vi "Create Task Taking XML.vi"(8 "error in (no error)":errorcluster) -> (0 "error out":errorcluster, 3 "Take Task XML":string)   [LabVIEW 2012]
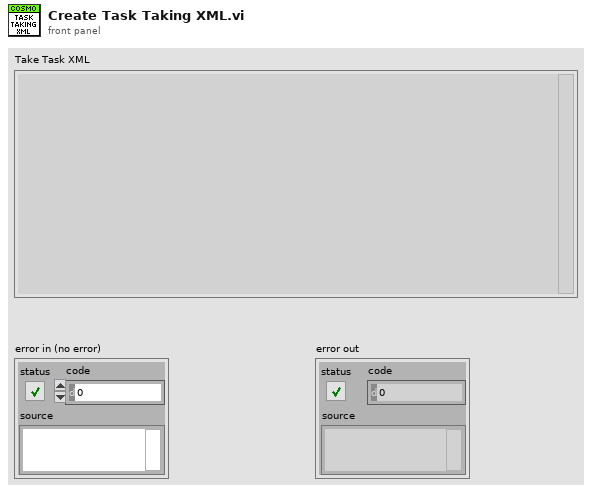
[diagram p1: front panel]
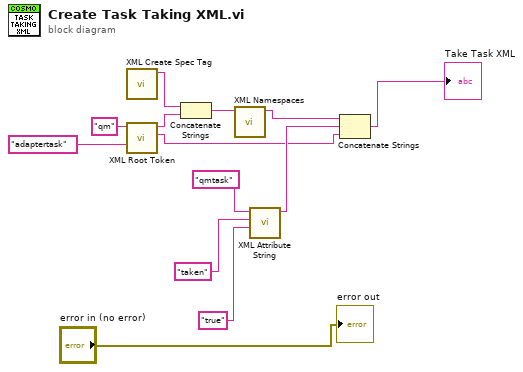
[diagram p0: block diagram]
diagram:
  n1 = call "XML Create Spec Tag.vi"() -> ("XML Spec tag"=w11:string)  [unwired: 11 in]
  n2 = call "XML Root Token.vi"("Tag"="adaptertask", "Namespace"="qm") -> ("Closing Item"=w2:string, "Root Item"=w10:string)  [unwired: 8 in]
  n3 = Concatenate Strings(w11, w10) -> (w9:string)
  n4 = call "XML Namespaces.vi"("String in"=w9) -> ("String out"=w5:string)  [unwired: 10 in]
  n5 = call "XML Attribute String.vi"("Value"="true", "Name"="taken" ("Prefix"), "Prefix"="qmtask") -> ("Attribute string"=w4:string)  [unwired: 8 in]
  n6 = Concatenate Strings(w5, w4, w2) -> (→"Take Task XML":string)
  "error out" <- "error in (no error)"
